vi "Initialize.vi"(0 "VISA resource name":refnum<visa-resource-name>, 5 "ID Query (T: Check)":bool=TRUE, 7 "Reset (T: Reset)":bool=TRUE, 11 "error in (no error)":errorcluster) -> (4 "VISA resource name out":refnum<visa-resource-name>, 15 "error out":errorcluster)   [LabVIEW 2020, in "Stanford Research PS300 Series.lvlib"]
doc: "This VI passes the addressing information in the instrument decriptor to the Instr Open VI and returns the instrument ID. You can optionally reset the instrument by setting the front panel reset control. You must run this VI before using any of the instrument driver VIs for this instrument."
uses:
  Stanford Research PS300 Series.lvlib
panel:
  # "(c) 2005-2015 National Instruments.  ALL RIGHTS RESERVED."
  # "Check\nDon't Check"
  # "Reset\nDon't Reset"
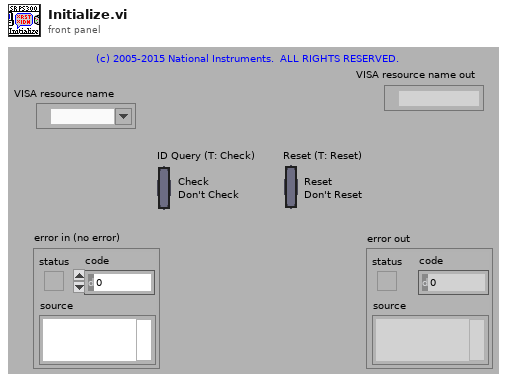
[diagram p1: front panel]
types:
  T1 = cluster{"status":bool, "code":i32, "VI Name":string}
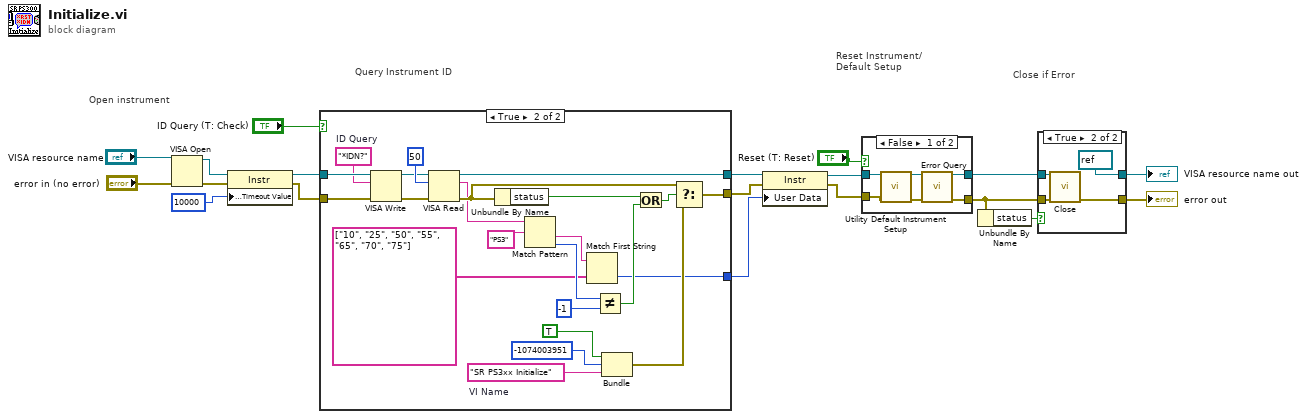
[diagram p0: block diagram]
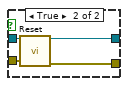
[diagram p3: hidden frame]
diagram:
  # "Close if Error"
  # "Query Instrument ID"
  # "Reset Instrument/\nDefault Setup"
  # "Open instrument"
  n1 = VISA Open(error in (no error)="error in (no error)", VISA resource name="VISA resource name") -> (VISA resource name=w10:refnum<visa-resource-name>, error out=w12:errorcluster)  [unwired: 3 in]
  n2 = property on="Property Node" class="Instr"(reference=w10, error in=w12, "General Settings:Timeout Value"=u32 10000 ("Tmo Value")) -> (reference out=w9:refnum<visa-resource-name>, error out=w11:errorcluster)
  n3 = case shown="True" "ID Query (T: Check)" {
    tunnel: [w21 w45] -> w4
    tunnel: [w22 w42] -> w5
    tunnel: w9 -> [w22 w43]
    tunnel: w11 -> [w21 w44]
    tunnel: [0 ("index") w23] -> w1
    frame False {
    }
    frame True {
      w38 = "*IDN?"  # ID Query
      w28 = "SR PS3xx Initialize"  # VI Name
      n4 = VISA Write(VISA resource name=w43, write buffer=w38, error in (no error)=w44) -> (VISA resource name out=w31:refnum<visa-resource-name>, error out=w33:errorcluster)  [unwired: 1 out]
      n5 = VISA Read(VISA resource name=w31, byte count=u32 50, error in (no error)=w33) -> (VISA resource name out=w42:refnum<visa-resource-name>, read buffer=w30:string, error out=w32:errorcluster)  [unwired: 1 out]
      n6 = Unbundle By Name(w32) -> ("status"=w35:bool)
      n7 = Match Pattern(string=w30, regular expression="PS3") -> (after substring=w25:string, offset past match=w27:i32)  [unwired: 1 in, 2 out]
      n8 = Match First String(2:string[] ["10", "25", "50", "55", "65", "70", "75"] ("string array"), 3:w25) -> (0:w23:i32)  [unwired: 1 out]
      n9 = Not Equal?(x=w27, y=-1) -> (x != y?=w29:bool)
      n10 = Bundle(TRUE, -1074003951, "VI Name"=w28) -> (w39:cluster{bool, i32, "VI Name":string})  [unwired: 1 in]
      n11 = Or(x=w35, y=w29) -> (x .or. y?=w34:bool)
      n12 = Select(t=w32, s=w34, f=w39) -> (s? t:f=w45:T1)
    }
  }
  n13 = property class="Instr"(reference=w5, error in=w4, "User Data"=w1) -> (reference out=w3:refnum<visa-resource-name>, error out=w2:errorcluster)
  n14 = case shown="False" "Reset (T: Reset)" {
    tunnel: w2 -> [w50 w52]
    tunnel: [w46 w55] -> w15
    tunnel: w3 -> [w51 w53]
    tunnel: [w47 w54] -> w14
    frame False {
      n15 = call "Utility Default Instrument Setup.vi"("VISA resource name"=w51, "error in (no error)"=w50) -> ("VISA resource name out"=w49:refnum<visa-resource-name>, "error out"=w48:errorcluster)  [unwired: 12 in]
      n16 = call "Error Query.vi"("VISA resource name"=w49, "error in (no error)"=w48) -> ("VISA resource name out"=w47:refnum<visa-resource-name>, "error out"=w46:errorcluster)  [unwired: 10 in, 2 out]
    }
    frame True {
      n17 = call "Reset.vi"("VISA resource name"=w53, "error in (no error)"=w52) -> ("VISA resource name out"=w54:refnum<visa-resource-name>, "error out"=w55:errorcluster)  [unwired: 12 in]
    }
  }
  n18 = Unbundle By Name(w15) -> ("status"=w16:bool)
  n19 = case shown="True" w16 {
    tunnel: w14 -> [w57 w60]
    tunnel: w15 -> [w56 w61]
    tunnel: [w57 refnum<visa-resource-name> refnum ("VISA resource name out")] -> w8
    tunnel: [w56 w59] -> w7
    frame False {
    }
    frame True {
      n20 = call "Close.vi"("VISA resource name"=w60, "error in (no error)"=w61) -> ("error out"=w59:errorcluster)  [unwired: 13 in]
    }
  }
  "VISA resource name out" <- w8
  "error out" <- w7
